vi "Initialize swept sine.vi"(1 "AO source settings":T6={"excitation channel"="", "max value [V]"=10.0, "min value [V]"=-10.0, "terminal configuration"=-1} {"terminal configuration" items=["Default"=-1, "RSE"=10083, "Differential"=10106, "Pseudodifferential"=12529]; "min value [V]" format="%0.2f"; "max value [V]" format="%0.2f"}, 2 "AI response settings":T5={"stimulus channel"="", "max value [V]"=10.0, "min value [V]"=-10.0, "terminal configuration"=-1} {"terminal configuration" items=["Default"=-1, "RSE"=10083, "NRSE"=10078, "Differential"=10106, "Pseudodifferential"=12529]; "min value [V]" format="%.2f"; "max value [V]" format="%.2f"}, 3 "error in (no error)":errorcluster) -> (7 "swept sine task out":T1={"source settings"={"AO task name"="", "source"=[]}, "stimulus settings"={"stimulus task name"="", "stimulus"=[]}, "response(s) settings"={"response task name"="", "response"=[]}, "measurement settings"={"AI sampling frequency"=51200.0, "AO sampling frequency"=1024.0, "AI block size"=1024, "AO block Size"=1024, "block duration [ms]"=0.0, "number of AI channels"=0, "device propagation delay [samples]"=0.0, "total propagation time [samples]"=0.0, "DUT propagation time [ms]"=0.0}, "linlog"=enum."linear", "repeat"=enum."off", "frequency list"=[1.0], "amplitude list"=[1.0], "settling time"={"settle time"=0.015599999576807022, "settle cycles"=5}, "integration time"={"integration time"=0.015599999576807022, "integration cycles"=5}, "frequencies indices"={"AI freq index"=0, "AO freq index"=5}, "read marks"={"write index"=0, "read index"=0, "freq start index"=0, "freq stop index"=0, "# extracted"=0, "buffer type"=enum."Invalid buffer", "read/write indices"=[], "AO index"=0, "AI index"=0, "settled"=FALSE, "integration done"=FALSE}, "harmonic settings"={"maximum THD harmonic"=5, "harmonic mapping"=[1], "units"={"THD unit"=enum."%", "nth harmonic unit"=enum."%", "SINAD unit"=enum."dB", "THD+N unit"=enum."dB"}}, "auto resolution settings"={"auto max step"=512, "slow threshold db"=6.0, "fast threshold db"=1.0}, "auto level settings"={"auto level enable"=FALSE, "auto level channel"=6, "ideal ref"=1.0, "max level"=10.0, "ref upper deviation db"=3.0, "ref lower deviation db"=-3.0}, "offset"=1.0, "ramping rate"=0.0, "phase"=0.0, "initialize"=FALSE} {"phase" format="%.2f"; "response(s) settings"."response"."channel info"."pregain" format="%.2f"; "response(s) settings"."response"."channel info"."weighting filter" items=["Linear", "A-weighting", "B-weighting", "C-weighting", "ITU-R 468-4", "Dolby", "CCITT", "C-message", "Wb", "Wc", "Wd", "We", "Wf", "Wh", "Wj", "Wk", "Wm", "AES17 20 kHz lowpass", "AES17 40 kHz lowpass", "AES17 20 kHz highpass", "AES17 40 kHz highpass"]; "response(s) settings"."response"."channel info"."dB reference" format="%^.1e"; "response(s) settings"."response"."channel info"."engineering units" items=["custom..."=0, "V"=1, "A"=21, "C"=30, "pC"=31, "s"=32, "-"=29, "Pa"=2, "N"=20, "g"=3, "m/s^2"=4, "m/s"=5, "m"=6, "mm/s"=12, "mm"=13, "micron/s"=14, "micron"=15, "in/s^2"=7, "in/s"=8, "in"=9, "mil/s"=10, "mil"=11, "rad/s^2"=16, "rad/s"=17, "rad"=18, "deg/s^2"=26, "deg/s"=27, "deg"=28, "RPM"=22, "cycle/s^2"=23, "Hz"=24, "cycle"=25, "strain"=19]; "response(s) settings"."response"."channel info"."sensor sensitivity" format="%#_5f"; "stimulus settings"."stimulus"."channel info"."pregain" format="%.2f"; "stimulus settings"."stimulus"."channel info"."weighting filter" items=["Linear", "A-weighting", "B-weighting", "C-weighting", "ITU-R 468-4", "Dolby", "CCITT", "C-message", "Wb", "Wc", "Wd", "We", "Wf", "Wh", "Wj", "Wk", "Wm", "AES17 20 kHz lowpass", "AES17 40 kHz lowpass", "AES17 20 kHz highpass", "AES17 40 kHz highpass"]; "stimulus settings"."stimulus"."channel info"."dB reference" format="%^.1e"; "stimulus settings"."stimulus"."channel info"."engineering units" items=["custom..."=0, "V"=1, "A"=21, "C"=30, "pC"=31, "s"=32, "-"=29, "Pa"=2, "N"=20, "g"=3, "m/s^2"=4, "m/s"=5, "m"=6, "mm/s"=12, "mm"=13, "micron/s"=14, "micron"=15, "in/s^2"=7, "in/s"=8, "in"=9, "mil/s"=10, "mil"=11, "rad/s^2"=16, "rad/s"=17, "rad"=18, "deg/s^2"=26, "deg/s"=27, "deg"=28, "RPM"=22, "cycle/s^2"=23, "Hz"=24, "cycle"=25, "strain"=19]; "stimulus settings"."stimulus"."channel info"."sensor sensitivity" format="%#_5f"; "ramping rate" format="%.4f"; "offset" format="%.2f"; "auto level settings"."ref lower deviation db" format="%.4f"; "auto level settings"."ref upper deviation db" format="%.4f"; "auto level settings"."max level" format="%.4f"; "auto level settings"."ideal ref" format="%.4f"; "auto resolution settings"."fast threshold db" format="%.4f"; "auto resolution settings"."slow threshold db" format="%.4f"; "harmonic settings"."maximum THD harmonic" max=10 step=1; "integration time"."integration time" format="%.2p"; "settling time"."settle time" format="%.2p"; "amplitude list" format="%.2f"; "frequency list" format="%.2f"; "measurement settings"."DUT propagation time [ms]" format="%.2f"; "measurement settings"."AO sampling frequency" format="%.2f"; "measurement settings"."AI sampling frequency" format="%.2f"}, 10 "error out":errorcluster)   [LabVIEW 2018]
uses:
  <vilib>/addons/Sound and Vibration/svt_Swept Sine/subVIs/sv_Swept Sine Task.ctl
  <vilib>/addons/_NISVFA/_Shared subVIs/Controls/svc_Channel Info.ctl
  <vilib>/addons/_NISVFA/_Shared subVIs/Controls/svc_Engineering Units Text Ring.ctl
  <vilib>/addons/_NISVFA/_Shared subVIs/Controls/svc_Weighting Filter Text Ring.ctl
  <vilib>/DAQmx/create/channels.llb/DAQmx Create Channel (AO-Voltage-Basic).vi
  <vilib>/DAQmx/create/channels.llb/DAQmx Create Channel (AI-Voltage-Basic).vi
  <resource>/objmgr/daqmx.rc
  <vilib>/addons/Sound and Vibration/svt_Swept Sine/SoundVib_SweptSine.lvlib
panel:
  in  "swept sine task default":T1={"source settings"={"AO task name"="", "source"=[]}, "stimulus settings"={"stimulus task name"="", "stimulus"=[]}, "response(s) settings"={"response task name"="", "response"=[]}, "measurement settings"={"AI sampling frequency"=51200.0, "AO sampling frequency"=51200.0, "AI block size"=1024, "AO block Size"=0, "block duration [ms]"=1024.0, "number of AI channels"=0, "device propagation delay [samples]"=0.0, "total propagation time [samples]"=0.0, "DUT propagation time [ms]"=0.0}, "linlog"=enum."linear", "repeat"=enum."off", "frequency list"=[1.0], "amplitude list"=[1.0], "settling time"={"settle time"=0.015599999576807022, "settle cycles"=5}, "integration time"={"integration time"=0.015599999576807022, "integration cycles"=5}, "frequencies indices"={"AI freq index"=0, "AO freq index"=0}, "read marks"={"write index"=0, "read index"=0, "freq start index"=0, "freq stop index"=0, "# extracted"=0, "buffer type"=enum."Invalid buffer", "read/write indices"=[], "AO index"=0, "AI index"=0, "settled"=FALSE, "integration done"=FALSE}, "harmonic settings"={"maximum THD harmonic"=5, "harmonic mapping"=[1], "units"={"THD unit"=enum."%", "nth harmonic unit"=enum."%", "SINAD unit"=enum."dB", "THD+N unit"=enum."dB"}}, "auto resolution settings"={"auto max step"=512, "slow threshold db"=6.0, "fast threshold db"=1.0}, "auto level settings"={"auto level enable"=FALSE, "auto level channel"=0, "ideal ref"=1.0, "max level"=10.0, "ref upper deviation db"=3.0, "ref lower deviation db"=-3.0}, "offset"=1.0, "ramping rate"=0.0, "phase"=0.0, "initialize"=FALSE} {"phase" format="%.2f"; "response(s) settings"."response"."channel info"."pregain" format="%.2f"; "response(s) settings"."response"."channel info"."weighting filter" items=["Linear", "A-weighting", "B-weighting", "C-weighting", "ITU-R 468-4", "Dolby", "CCITT", "C-message", "Wb", "Wc", "Wd", "We", "Wf", "Wh", "Wj", "Wk", "Wm", "AES17 20 kHz lowpass", "AES17 40 kHz lowpass", "AES17 20 kHz highpass", "AES17 40 kHz highpass"]; "response(s) settings"."response"."channel info"."dB reference" format="%^.1e"; "response(s) settings"."response"."channel info"."engineering units" items=["custom..."=0, "V"=1, "A"=21, "C"=30, "pC"=31, "s"=32, "-"=29, "Pa"=2, "N"=20, "g"=3, "m/s^2"=4, "m/s"=5, "m"=6, "mm/s"=12, "mm"=13, "micron/s"=14, "micron"=15, "in/s^2"=7, "in/s"=8, "in"=9, "mil/s"=10, "mil"=11, "rad/s^2"=16, "rad/s"=17, "rad"=18, "deg/s^2"=26, "deg/s"=27, "deg"=28, "RPM"=22, "cycle/s^2"=23, "Hz"=24, "cycle"=25, "strain"=19]; "response(s) settings"."response"."channel info"."sensor sensitivity" format="%#_5f"; "stimulus settings"."stimulus"."channel info"."pregain" format="%.2f"; "stimulus settings"."stimulus"."channel info"."weighting filter" items=["Linear", "A-weighting", "B-weighting", "C-weighting", "ITU-R 468-4", "Dolby", "CCITT", "C-message", "Wb", "Wc", "Wd", "We", "Wf", "Wh", "Wj", "Wk", "Wm", "AES17 20 kHz lowpass", "AES17 40 kHz lowpass", "AES17 20 kHz highpass", "AES17 40 kHz highpass"]; "stimulus settings"."stimulus"."channel info"."dB reference" format="%^.1e"; "stimulus settings"."stimulus"."channel info"."engineering units" items=["custom..."=0, "V"=1, "A"=21, "C"=30, "pC"=31, "s"=32, "-"=29, "Pa"=2, "N"=20, "g"=3, "m/s^2"=4, "m/s"=5, "m"=6, "mm/s"=12, "mm"=13, "micron/s"=14, "micron"=15, "in/s^2"=7, "in/s"=8, "in"=9, "mil/s"=10, "mil"=11, "rad/s^2"=16, "rad/s"=17, "rad"=18, "deg/s^2"=26, "deg/s"=27, "deg"=28, "RPM"=22, "cycle/s^2"=23, "Hz"=24, "cycle"=25, "strain"=19]; "stimulus settings"."stimulus"."channel info"."sensor sensitivity" format="%#_5f"; "ramping rate" format="%.4f"; "offset" format="%.2f"; "auto level settings"."ref lower deviation db" format="%.4f"; "auto level settings"."ref upper deviation db" format="%.4f"; "auto level settings"."max level" format="%.4f"; "auto level settings"."ideal ref" format="%.4f"; "auto resolution settings"."fast threshold db" format="%.4f"; "auto resolution settings"."slow threshold db" format="%.4f"; "harmonic settings"."maximum THD harmonic" max=10 step=1; "integration time"."integration time" format="%.2p"; "settling time"."settle time" format="%.2p"; "amplitude list" format="%.2f"; "frequency list" format="%.2f"; "measurement settings"."DUT propagation time [ms]" format="%.2f"; "measurement settings"."AO sampling frequency" format="%.2f"; "measurement settings"."AI sampling frequency" format="%.2f"}
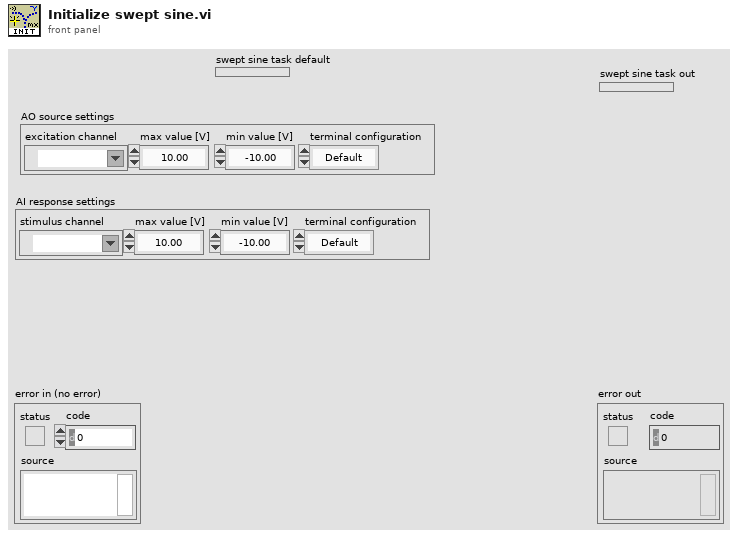
[diagram p1: front panel]
types:
  T1 = typedef "SoundVib_SweptSine.lvlib/sv_Swept Sine Task.ctl" = cluster{"source settings":cluster{"AO task name":refnum<k21>, "source":cluster{"AO physical channel":tag}[]}, "stimulus settings":cluster{"stimulus task name":refnum<k21>, "stimulus":cluster{"stimulus physical channel":tag, "channel info":T2}[]}, "response(s) settings":cluster{"response task name":refnum<k21>, "response":cluster{"response physical channel":tag, "channel info":T2}[]}, "measurement settings":cluster{"AI sampling frequency":dbl, "AO sampling frequency":dbl, "AI block size":i32, "AO block Size":i32, "block duration [ms]":dbl, "number of AI channels":i32, "device propagation delay [samples]":dbl, "total propagation time [samples]":dbl, "DUT propagation time [ms]":dbl}, "linlog":enum16{"linear", "log"}, "repeat":enum16{"off", "on"}, "frequency list":dbl[], "amplitude list":dbl[], "settling time":cluster{"settle time":dbl, "settle cycles":i32}, "integration time":cluster{"integration time":dbl, "integration cycles":i32}, "frequencies indices":cluster{"AI freq index":i32, "AO freq index":i32}, "read marks":cluster{"write index":u32, "read index":u32, "freq start index":u32, "freq stop index":u32, "# extracted":u32, "buffer type":enum16{"Invalid buffer", "Intermediate buffer", "Final buffer"}, "read/write indices":cluster{"settle time index":u32, "integration time index":u32}[], "AO index":i32, "AI index":i32, "settled":bool, "integration done":bool}, "harmonic settings":cluster{"maximum THD harmonic":u32, "harmonic mapping":u32[], "units":cluster{"THD unit":enum16{"dB", "%"}, "nth harmonic unit":enum16{"dB", "%"}, "SINAD unit":enum16{"dB", "%"}, "THD+N unit":enum16{"dB", "%"}}}, "auto resolution settings":cluster{"auto max step":i32, "slow threshold db":dbl, "fast threshold db":dbl}, "auto level settings":cluster{"auto level enable":bool, "auto level channel":u8, "ideal ref":sgl, "max level":sgl, "ref upper deviation db":sgl, "ref lower deviation db":sgl}, "offset":dbl, "ramping rate":dbl, "phase":dbl, "initialize":bool}
  T2 = typedef "svc_Channel Info.ctl" = cluster{"sensor sensitivity":dbl, "engineering units":T3, "dB reference":dbl, "custom label":string, "weighting filter":T4, "pregain":dbl}
  T3 = typedef "svc_Engineering Units Text Ring.ctl" = u16
  T4 = typedef "svc_Weighting Filter Text Ring.ctl" = u16
  T5 = cluster{"stimulus channel":tag, "max value [V]":dbl, "min value [V]":dbl, "terminal configuration":i32}
  T6 = cluster{"excitation channel":tag, "max value [V]":dbl, "min value [V]":dbl, "terminal configuration":i32}
  T7 = cluster{"settle time index":u32, "integration time index":u32}[]
  T8 = enum16{"Invalid buffer", "Intermediate buffer", "Final buffer"}
  T9 = cluster{"DAQmx Physical Channel":tag, "channel info":T2}
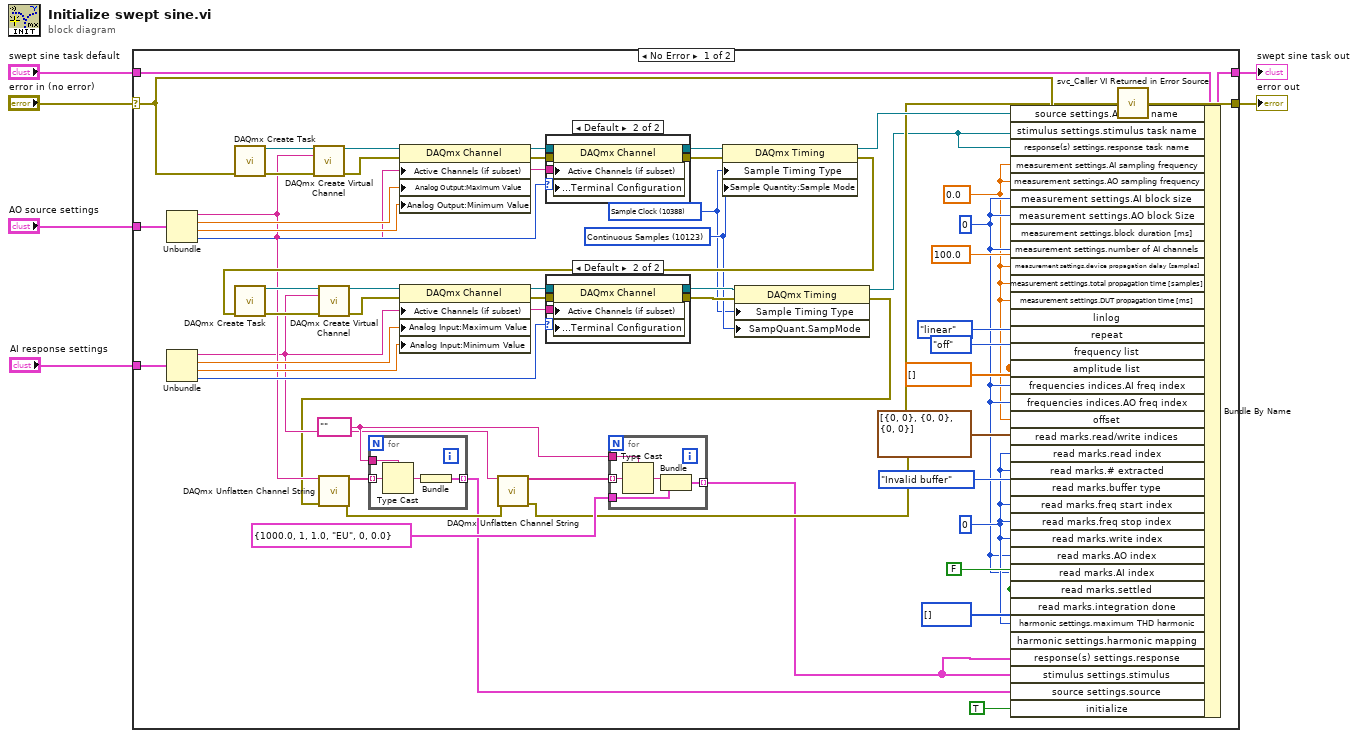
[diagram p0: block diagram]
diagram:
  n1 = case shown="No Error" "error in (no error)" {
    selector: "error in (no error)" -> [w18 w89]
    tunnel: [w55 w89] -> w6
    tunnel: [w52 w88] -> w5
    tunnel: "AO source settings" -> [w45 _]
    tunnel: "AI response settings" -> [w47 _]
    tunnel: "swept sine task default" -> [w54 w88]
    frame No Error {
      w60 = dbl[] [] ("frequency list")
      w29 = 0.0 ("measurement settings.AI sampling frequency")
      w10 = 10123 items=["Finite Samples"=10178, "Continuous Samples"=10123, "Hardware Timed Single Point"=12522] ("SampQuant.SampMode")
      w9 = 10388 items=["Sample Clock"=10388, "Handshake"=10389, "Implicit"=10451, "On Demand"=10390, "Change Detection"=12504] ("SampTimingType")
      w31 = 0 ("AO device settings.AO Settings.AO taskID")
      w34 = tag "" ("DAQmx Physical Channel")
      w58 = FALSE ("acq state.settled")
      w53 = u32 0 ("AO device settings.AO Settings.AO taskID")
      n2 = Unbundle(w45) -> ("excitation channel"=w17:tag, "max value [V]"=w42:dbl, "min value [V]"=w41:dbl, "terminal configuration"=w25:i32)
      n3 = Unbundle(w47) -> ("stimulus channel"=w16:tag, "max value [V]"=w46:dbl, "min value [V]"=w48:dbl, "terminal configuration"=w24:i32)
      n4 = call <vilib>:"DAQmx Create Task.vi"("error in"=w18) -> ("task out"=w51:refnum<k21>, "error out"=w36:errorcluster)  [unwired: 13 in]
      n5 = call-poly <vilib>:"DAQmx Create Virtual Channel.vi"("task in"=w51, "physical channels"=w17, "error in"=w36) -> ("task out"=w44:refnum<k21>, "error out"=w43:errorcluster)  [unwired: 11 in]
      n6 = property class="DAQmx Channel"(reference=w44, error in=w43, "Active Channels (if subset)"=w17, "Analog Output:Maximum Value"=w42, "Analog Output:Minimum Value"=w41) -> (reference out=w28:refnum<k21>, error out=w27:errorcluster)
      n7 = case shown="Default" w25 {
        selector: w25 -> [_ w73]
        tunnel: w28 -> [w72 w78]
        tunnel: w27 -> [w71 w77]
        tunnel: [w72 w76] -> w22
        tunnel: w17 -> [_ w75]
        tunnel: [w71 w74] -> w20
        frame -1 {
          # "Use default:\nterminal config"
        }
        frame Default {
          n8 = property class="DAQmx Channel"(reference=w78, error in=w77, "Active Channels (if subset)"=w75, "Analog Output:General Properties:Output Configuration:Terminal Configuration"=w73) -> (reference out=w76:refnum<k21>, error out=w74:errorcluster)
        }
      }
      n9 = property class="DAQmx Timing"(reference=w22, error in=w20, "Sample Timing Type"=w9, "Sample Quantity:Sample Mode"=w10) -> (reference out=w23:refnum<k21>, error out=w21:errorcluster)
      n10 = call <vilib>:"DAQmx Create Task.vi"("error in"=w21) -> ("task out"=w33:refnum<k21>, "error out"=w35:errorcluster)  [unwired: 13 in]
      n11 = call-poly <vilib>:"DAQmx Create Virtual Channel.vi"("task in"=w33, "physical channels"=w16, "error in"=w35) -> ("task out"=w49:refnum<k21>, "error out"=w50:errorcluster)  [unwired: 11 in]
      n12 = property class="DAQmx Channel"(reference=w49, error in=w50, "Active Channels (if subset)"=w16, "Analog Input:Maximum Value"=w46, "Analog Input:Minimum Value"=w48) -> (reference out=w26:refnum<k21>, error out=w15:errorcluster)
      n13 = case shown="Default" w24 {
        selector: w24 -> [_ w65]
        tunnel: w26 -> [w64 w70]
        tunnel: w15 -> [w63 w69]
        tunnel: [w64 w68] -> w12
        tunnel: w16 -> [_ w67]
        tunnel: [w63 w66] -> w13
        frame -1 {
          # "Use default:\nterminal config"
        }
        frame Default {
          n14 = property class="DAQmx Channel"(reference=w70, error in=w69, "Active Channels (if subset)"=w67, "Analog Input:General Properties:Input Configuration:Terminal Configuration"=w65) -> (reference out=w68:refnum<k21>, error out=w66:errorcluster)
        }
      }
      n15 = property class="DAQmx Timing"(reference=w12, error in=w13, "Sample Timing Type"=w9, "SampQuant.SampMode"=w10) -> (reference out=w7:refnum<k21>, error out=w11:errorcluster)
      n16 = call <vilib>:"DAQmx Unflatten Channel String.vi"("names in"=w17, "error in"=w11) -> ("names out"=w40:string[], "error out"=w32:errorcluster)  [unwired: 12 in]
      n17 = for {
        tunnel: w40 -> [w86] mode=indexing
        tunnel: [w87] -> w30 mode=indexing
        tunnel: w34 -> [w84]
        n18 = Type Cast(type=w84, x=w86) -> (*(type *) &x=w85:tag)
        n19 = Bundle("DAQmx Physical Channel"=w85) -> (w87:cluster{"DAQmx Physical Channel":tag})  [unwired: 1 in]
      }
      n20 = call <vilib>:"DAQmx Unflatten Channel String.vi"("names in"=w16, "error in"=w32) -> ("names out"=w39:string[], "error out"=w14:errorcluster)  [unwired: 12 in]
      n21 = for {
        tunnel: w39 -> [w82] mode=indexing
        tunnel: [w83] -> w8 mode=indexing
        tunnel: w34 -> [w80]
        tunnel: T2 {"sensor sensitivity"=1000.0, "engineering units"=1, "dB reference"=1.0, "custom label"="EU", "weighting filter"=0, "pregain"=0.0} ("channel info") -> [w79]
        n22 = Type Cast(type=w80, x=w82) -> (*(type *) &x=w81:tag)
        n23 = Bundle("DAQmx Physical Channel"=w81, "channel info"=w79) -> (w83:T9)  [unwired: 1 in]
      }
      n24 = Bundle By Name(cluster=w54, "source settings.AO task name"=w23, "stimulus settings.stimulus task name"=w7, "response(s) settings.response task name"=w7, "measurement settings.AI sampling frequency"=w29, "measurement settings.AO sampling frequency"=w29, "measurement settings.AI block size"=w31, "measurement settings.AO block Size"=w31, "measurement settings.block duration [ms]"=100.0, "measurement settings.number of AI channels"=w31, "measurement settings.device propagation delay [samples]"=w29, "measurement settings.total propagation time [samples]"=w29, "measurement settings.DUT propagation time [ms]"=w29, "linlog"=enum16{"linear", "log"}."linear", "repeat"=enum16{"off", "on"}."off", "frequency list"=w60, "amplitude list"=w60, "frequencies indices.AI freq index"=w31, "frequencies indices.AO freq index"=w31, "offset"=w29, "read marks.read/write indices"=T7 [{"settle time index"=0, "integration time index"=0}, {"settle time index"=0, "integration time index"=0}, {"settle time index"=0, "integration time index"=0}] ("initialized array"), "read marks.read index"=w53, "read marks.# extracted"=w53, "read marks.buffer type"=T8."Invalid buffer", "read marks.freq start index"=w53, "read marks.freq stop index"=w53, "read marks.write index"=w53, "read marks.AO index"=w31, "read marks.AI index"=w31, "read marks.settled"=w58, "read marks.integration done"=w58, "harmonic settings.maximum THD harmonic"=w53, "harmonic settings.harmonic mapping"=u32[] [], "response(s) settings.response"=w8, "stimulus settings.stimulus"=w8, "source settings.source"=w30, "initialize"=TRUE) -> (w52:T1)
      n25 = call <vilib>:"svc_Caller VI Returned in Error Source.vi"("warning input to caller"=w18, "error in (no error)"=w14) -> ("error out"=w55:errorcluster)  [unwired: 3 in]
    }
    frame Error {
    }
  }
  "error out" <- w6
  "swept sine task out" <- w5
